vi "Check and Apply VIPC.vi"(8 "error in (no error)":errorcluster, 11 "VIPC File Path":path) -> (0 "error out":errorcluster)   [LabVIEW 2014]
uses:
  <userlib>/_OpenG.lib/file/file.llb/File Exists - Scalar__ogtk.vi
  <vilib>/JKI/VIPM API/VIPM API_vipm_api.lvlib
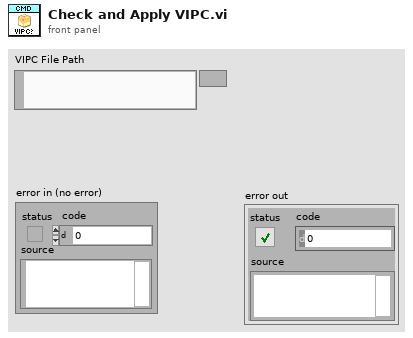
[diagram p1: front panel]
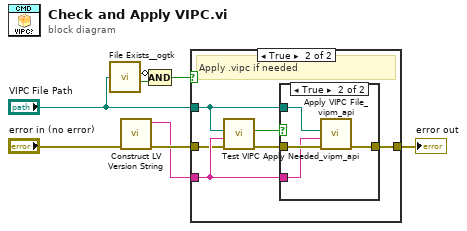
[diagram p0: block diagram]
diagram:
  n1 = call-poly <userlib>:"File Exists__ogtk.vi"("file path"="VIPC File Path") -> ("is directory"=w6:bool, "exists"=w5:bool)  [unwired: 6 in]
  n2 = call "Construct LV Version String.vi"("error in (no error)"="error in (no error)") -> ("error out"=w2:errorcluster, "LabVIEW Version"=w1:string)  [unwired: 9 in]
  n3 = Compound Arithmetic op=AND(invert w6, w5) -> (w4:bool)
  n4 = case shown="True" w4 {
    tunnel: "VIPC File Path" -> [_ w13]
    tunnel: [w9 w12] -> w8
    tunnel: w1 -> [_ w11]
    tunnel: w2 -> [w9 w10]
    frame False {
      # "Allow missing .vipc for now"
    }
    frame True {
      # "Apply .vipc if needed"
      n5 = call <vilib>:"Test VIPC Apply Needed_vipm_api.vi"("error in (no error)"=w10, "LabVIEW Version (use vipc version)"=w11, "VIPC File Path"=w13) -> ("error out"=w14:errorcluster, "Need to Apply?"=w15:bool)  [unwired: 7 in]
      n6 = case shown="True" w15 {
        tunnel: w14 -> [w16 w20]
        tunnel: w13 -> [_ w19]
        tunnel: [w16 w18] -> w12
        tunnel: w11 -> [_ w17]
        frame False {
        }
        frame True {
          n7 = call <vilib>:"Apply VIPC File_vipm_api.vi"("error in (no error)"=w20, "LabVIEW Version"=w17, "VIPC File"=w19) -> ("error out"=w18:errorcluster)  [unwired: 8 in]
        }
      }
    }
  }
  "error out" <- w8
